vi "PID Geschwin (SubVI).vi"(0 "lower limit":dbl format="%0.2f", 2 "Rück Geschwin":dbl, 3 "upper limit":dbl format="%0.2f", 4 "Kp Geschwin":dbl, 5 "Ki Geschwin":dbl, 6 "D":dbl=0.05 format="%0.2f", 7 "Führung Geschwin":dbl) -> (1 "OUT Gesch":dbl)   [LabVIEW 2010]
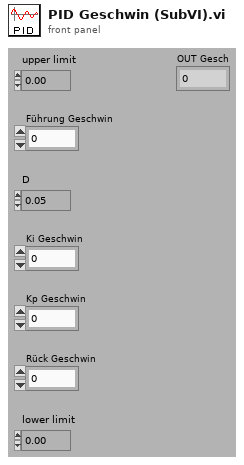
[diagram p1: front panel]
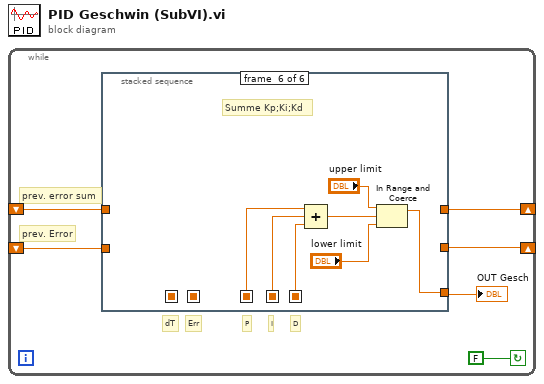
[diagram p0: block diagram]
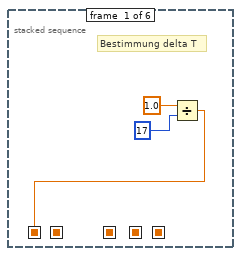
[diagram p2: hidden frame]
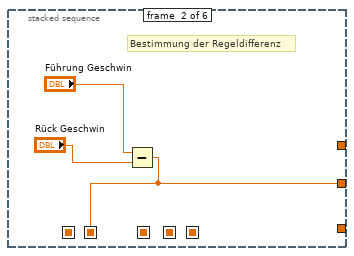
[diagram p3: hidden frame]
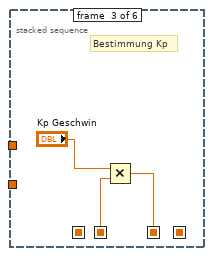
[diagram p4: hidden frame]
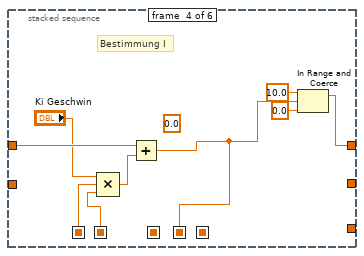
[diagram p5: hidden frame]
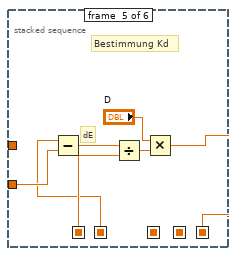
[diagram p6: hidden frame]
diagram:
  n1 = while {
    shift-left: _ -> [w3]
    shift-right: [w4] -> _
    shift-left: _ -> [w6]
    shift-right: [w5] -> _
    stop <- FALSE continue-if-true
    # "I"
    # "dT"
    # "Err"
    # "D"
    # "P"
    # "prev. error sum"
    # "prev. Error"
    n2 = stacked-sequence {
      seq-local: [w8 _ _ _ _ _] -> [_ _ _ w22 w28 _]
      seq-local: [_ w12 _ _ _ _] -> [_ _ w15 w21 w27 _]
      seq-local: [_ _ w14 _ _ _] -> [_ _ _ _ _ w37]
      seq-local: [_ _ _ _ w25 _] -> [_ _ _ _ _ w35]
      seq-local: [_ _ _ w16 _ _] -> [_ _ _ _ _ w36]
      tunnel: w6 -> [_ _ _ w23 _ _]
      tunnel: [_ _ _ w19 _ _] -> w5
      tunnel: [_ w12 _ _ _ _] -> w4
      tunnel: w3 -> [_ _ _ _ w29 _]
      tunnel: [_ _ _ _ _ w34] -> w1
      frame #0 {
        # "Bestimmung delta T"
        n3 = Divide(x=1.0, y=17) -> (x/y=w8:dbl)
      }
      frame #1 {
        # "Bestimmung der Regeldifferenz"
        n4 = Subtract(x="Führung Geschwin", y="Rück Geschwin") -> (x-y=w12:dbl)
      }
      frame #2 {
        # "Bestimmung Kp"
        n5 = Multiply(x="Kp Geschwin", y=w15) -> (x*y=w14:dbl)
      }
      frame #3 {
        (unwired) 0.0 ("t")
        # "Bestimmung I"
        n6 = Compound Arithmetic op=MULTIPLY("Ki Geschwin", w22, w21) -> (w24:dbl)
        n7 = Add(x=w23, y=w24) -> (x+y=w16:dbl)
        n8 = In Range and Coerce(upper limit=10.0 ("Obergrenze"), x=w16, lower limit=0.0 ("Untergrenze")) -> (coerced(x)=w19:dbl)  [unwired: 1 out]
      }
      frame #4 {
        # "dE"
        # "Bestimmung Kd"
        n9 = Subtract(x=w27, y=w29) -> (x-y=w30:dbl)
        n10 = Divide(x=w30, y=w28) -> (x/y=w31:dbl)
        n11 = Multiply(x="D", y=w31) -> (x*y=w25:dbl)
      }
      frame #5 {
        # "Summe Kp;Ki;Kd"
        n12 = Compound Arithmetic op=ADD(w37, w36, w35) -> (w38:dbl)
        n13 = In Range and Coerce(upper limit="upper limit", x=w38, lower limit="lower limit") -> (coerced(x)=w34:dbl)  [unwired: 1 out]
      }
    }
    "OUT Gesch" <- w1
  }
